vi "IR LIDAR.vi"() -> (0 "error out":errorcluster, 3 "Range":T1)   [LabVIEW 2014]
uses:
  <vilib>/myRIO/Instrument Drivers/Onboard IO/AI/typedefs/AI Reference.ctl
  <vilib>/myRIO/Common/Instrument Driver Framework/Utilities/typedefs/myRIO Generic Hardware Reference.ctl
  <vilib>/myRIO/Common/Instrument Driver Framework/Utilities/typedefs/Hardware Version Enum.ctl
  <vilib>/myRIO/Common/Instrument Driver Framework/Utilities/typedefs/myRIO v1.0 Reference.ctl
  <vilib>/myRIO/Common/Instrument Driver Framework/Utilities/typedefs/Generic FPGA Reference.ctl
  <vilib>/myRIO/Common/Instrument Driver Framework/myRIO v1.0/AI/typedefs/AI Channels List.ctl
  <vilib>/myRIO/Common/Instrument Driver Framework/myRIO v1.0/AI/typedefs/AI Channels Enum.ctl
  <vilib>/myRIO/Common/Instrument Driver Framework/Utilities/typedefs/Analog Scaling Constants List.ctl
  <vilib>/myRIO/Common/Instrument Driver Framework/Utilities/typedefs/Analog Scaling Constants.ctl
  <vilib>/userdefined/High Color/nirio_resource_hc.ctl
  <vilib>/myRIO/Common/Instrument Driver Framework/Utilities/vis/Is FPGA Ref Available.vi
  <vilib>/myRIO/Common/Instrument Driver Framework/myRIO v1.0/AI/vis/myRIO v1.1 Open AI.vi
  <vilib>/myRIO/Instrument Drivers/Onboard IO/AI/vis/Read.vi
  <vilib>/myRIO/Common/Instrument Driver Framework/Utilities/vis/Validate Channels.vi
  <vilib>/myRIO/Common/Instrument Driver Framework/myRIO v1.0/AI/vis/myRIO v1.0 Reserve AI.vi
  <vilib>/myRIO/Common/Instrument Driver Framework/myRIO v1.0/AI/vis/myRIO v1.0 Build MUX Configuration AI.vi
  <vilib>/myRIO/Common/Instrument Driver Framework/myRIO v1.0/Resource Manager/vis/myRIO v1.0 Reserve Channel List.vi
  <vilib>/myRIO/Common/Instrument Driver Framework/myRIO v1.0/Resource Manager/vis/myRIO v1.0 Reserve Channel.vi
  <vilib>/myRIO/Common/Instrument Driver Framework/myRIO v1.0/Resource Manager/vis/myRIO v1.0 Unreserve Channel.vi
  <vilib>/myRIO/Common/Instrument Driver Framework/myRIO v1.0/Resource Manager/vis/myRIO v1.0 Build Mutex Name.vi
  <vilib>/Utility/VariantDataType/GetNumericInfo.vi
  <vilib>/Utility/error.llb/Error Cluster From Error Code.vi
  <vilib>/myRIO/Common/Instrument Driver Framework/myRIO v1.0/myRIO v1.1 Open.vi
  <vilib>/myRIO/Common/Instrument Driver Framework/myRIO v1.0/AI/vis/myRIO v1.0 Get Scaling Constants AI.vi
  <vilib>/myRIO/Common/Instrument Driver Framework/Utilities/vis/IO Manager.vi
  <vilib>/myRIO/Common/Instrument Driver Framework/Utilities/vis/Configuration Manager.vi
  <vilib>/myRIO/Common/Instrument Driver Framework/myRIO v1.0/myRIO v1.0 Close.vi
  <vilib>/myRIO/Common/Instrument Driver Framework/myRIO v1.0/AI/vis/myRIO v1.0 Read AI.vi
  <vilib>/myRIO/Express VI/Onboard IO/AI/AI Express VI.xnode
  <vilib>/myRIO/Instrument Drivers/Onboard IO/AI/vis/myRIO AI Open.xnode
  <vilib>/myRIO/Instrument Drivers/Onboard IO/AI/AI.lvlib
panel:
  # "This subVI reads and \ncalibrates the three\nSharp IR\nrange sensor"
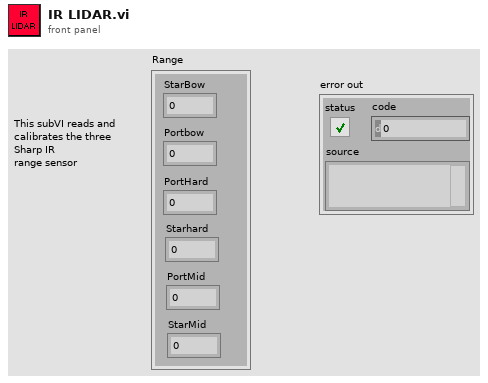
[diagram p1: front panel]
types:
  T1 = cluster{"StarBow":dbl, "Portbow":dbl, "PortHard":dbl, "Starhard":dbl, "PortMid":dbl, "StarMid":dbl}
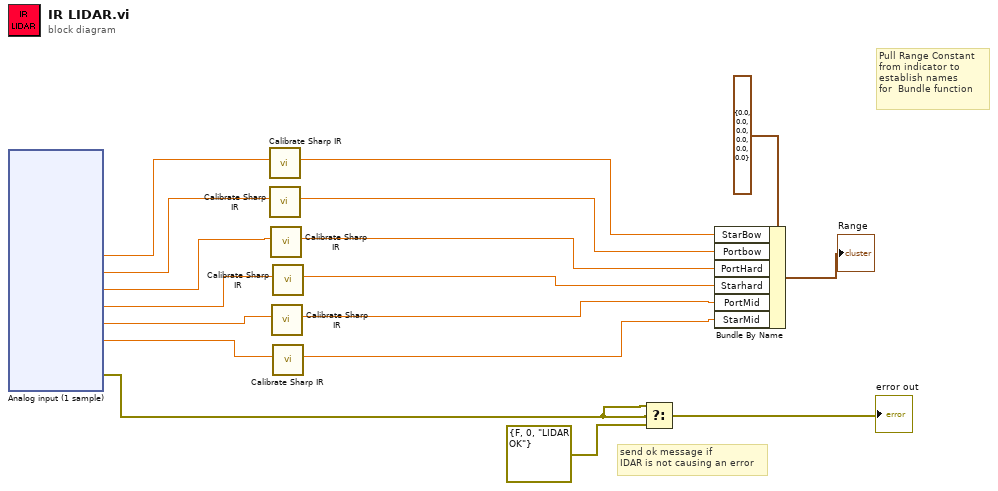
[diagram p0: block diagram]
diagram:
  # "Pull Range Constant\nfrom indicator to\nestablish names\nfor  Bundle function"
  # "send ok message if\nIDAR is not causing an error"
  n1 = xnode "Analog input (1 sample)"() -> ("StarBow (A/AI0 (Pin 3))"=w12:dbl, "PortBow (A/AI1 (Pin 5))"=w11:dbl, "PortHard (A/AI2 (Pin 7))"=w10:dbl, "StarHard (A/AI3 (Pin 9))"=w9:dbl, "PortMid (B/AI0 (Pin 3))"=w8:dbl, "StarMid (B/AI1 (Pin 5))"=w7:dbl, "error out"=w17:errorcluster)  [unwired: 1 in]
  n2 = call "Calibrate Sharp IR.vi"("IR Raw In"=w12) -> ("IR Calibrated Out"=w6:dbl)  [unwired: 10 in]
  n3 = call "Calibrate Sharp IR.vi"("IR Raw In"=w11) -> ("IR Calibrated Out"=w5:dbl)  [unwired: 10 in]
  n4 = call "Calibrate Sharp IR.vi"("IR Raw In"=w10) -> ("IR Calibrated Out"=w4:dbl)  [unwired: 10 in]
  n5 = call "Calibrate Sharp IR.vi"("IR Raw In"=w8) -> ("IR Calibrated Out"=w2:dbl)  [unwired: 10 in]
  n6 = call "Calibrate Sharp IR.vi"("IR Raw In"=w9) -> ("IR Calibrated Out"=w3:dbl)  [unwired: 10 in]
  n7 = call "Calibrate Sharp IR.vi"("IR Raw In"=w7) -> ("IR Calibrated Out"=w1:dbl)  [unwired: 10 in]
  n8 = Select(t=w17, s=w17, f=errorcluster {"status"=FALSE, "code"=0, "source"="LIDAR OK"} ("error out")) -> (s? t:f=→"error out":errorcluster)
  n9 = Bundle By Name "Bundle By Name"(cluster=T1 {"StarBow"=0.0, "Portbow"=0.0, "PortHard"=0.0, "Starhard"=0.0, "PortMid"=0.0, "StarMid"=0.0} ("Range"), "StarBow"=w6, "Portbow"=w5, "PortHard"=w4, "Starhard"=w3, "PortMid"=w2, "StarMid"=w1) -> (→"Range":T1)
